vi "Initialize.vi"(8 "error in":errorcluster, 10 "InstanceName":string, 11 "Cycler Cluster - 24 Channel.lvclass":refnum<class "Cycler Cluster - 6 Channel.lvclass">) -> (0 "error out":errorcluster, 3 "output cluster":refnum<class "Cycler Cluster - 6 Channel.lvclass">)   [LabVIEW 2023, in "Cycler Cluster - 6 Channel.lvclass"]
uses:
  Cycler Cluster - 6 Channel.lvclass
  Cycler Cluster - 6 Channel.lvclass/Cycler Cluster - 6 Channel.ctl
  7d45be24-9a40-4f36-b3d1-14bc4134107c.vi
  1abf7531-339f-4e14-8fbe-02c4e44e8943.vi
  da48c8f8-b897-4dcf-9451-5b341042a248.vi
  f0f9fcd1-ad99-4552-afb1-31be6853704b.vi
  7d45be24-9a40-4f36-b3d1-14bc4134107c.vi/4bc1c15b-36ab-481f-b8dd-c64075ce723a.vi
  1abf7531-339f-4e14-8fbe-02c4e44e8943.vi/4bc1c15b-36ab-481f-b8dd-c64075ce723a.vi
  da48c8f8-b897-4dcf-9451-5b341042a248.vi/4bc1c15b-36ab-481f-b8dd-c64075ce723a.vi
  f0f9fcd1-ad99-4552-afb1-31be6853704b.vi/4bc1c15b-36ab-481f-b8dd-c64075ce723a.vi
  <vilib>/ADAS Replay HIL/AdasHilServices/AdasHilServices Fill In Error Info Ex.vi
  Utilities/Utilities.lvlib
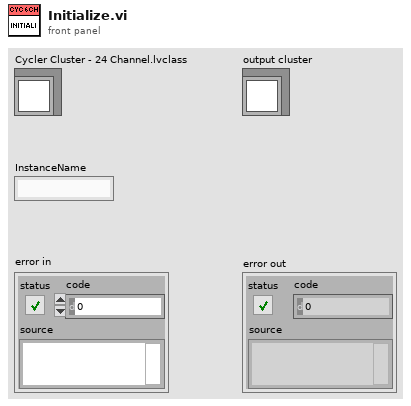
[diagram p1: front panel]
types:
  T1 = cluster{"OnOff.ACT":bool, "ErrorAcknowledge.ACT":bool, "IsoMeasurement.ACT":bool, "ParallelMode.ACT":bool}
  T2 = cluster{"OnOff.STS":i32, "Error.STS":i32, "Watchdog.STS":i32, "IsoMeasurement.STS":i32, "ParallelMode.STS":i32}
  T3 = cluster{"ErrorAcknowledge.ch01.ACT":bool, "OutputEnable.ch01.ACT":bool, "ControlMode.ch01.CTL":u16, "Voltage.ch01.SP":dbl, "VoltageMIN.ch01.SP":dbl, "VoltageMAX.ch01.SP":dbl, "VoltageGrad.ch01.SP":dbl, "Current.ch01.SP":dbl, "CurrentMIN.ch01.SP":dbl, "CurrentMAX.ch01.SP":dbl, "CurrentGrad.ch01.SP":dbl, "Power.ch01.SP":dbl, "Power.ch01.SP":dbl, "Power.ch01.SP":dbl, "PowerGrad.ch01.SP":dbl, "ParameterSet.ch01.CTL":i32}
  T4 = cluster{"Error.ch01.STS":i32, "OutputEnable.ch01.STS":i32, "ControlMode.ch01.STS":u16, "Voltage.ch01.AV":dbl, "Current.ch01.AV":dbl, "Power.ch01.AV":dbl, "VoltageNominal.ch01.AV":dbl, "CurrentNominal.ch01.AV":dbl, "PowerNominal.ch01.AV":dbl, "ParameterSet.ch01.STS":i32}
  T5 = cluster{"ErrorAcknowledge.ch02.ACT":bool, "OutputEnable.ch02.ACT":bool, "ControlMode.ch02.CTL":u16, "Voltage.ch02.SP":dbl, "VoltageMIN.ch02.SP":dbl, "VoltageMAX.ch02.SP":dbl, "VoltageGrad.ch02.SP":dbl, "Current.ch02.SP":dbl, "CurrentMIN.ch02.SP":dbl, "CurrentMAX.ch02.SP":dbl, "CurrentGrad.ch02.SP":dbl, "Power.ch02.SP":dbl, "PowerMIN.ch02.SP":dbl, "PowerMAX.ch02.SP":dbl, "PowerGrad.ch02.SP":dbl, "ParameterSet.ch02.CTL":i32}
  T6 = cluster{"Error.ch02.STS":i32, "OutputEnable.ch02.STS":i32, "ControlMode.ch02.STS":u16, "Voltage.ch02.AV":dbl, "Current.ch02.AV":dbl, "Power.ch02.AV":dbl, "VoltageNominal.ch02.AV":dbl, "CurrentNominal.ch02.AV":dbl, "PowerNominal.ch02.AV":dbl, "ParameterSet.ch02.STS":i32}
  T7 = cluster{"ErrorAcknowledge.ch03.ACT":bool, "OutputEnable.ch03.ACT":bool, "ControlMode.ch03.CTL":u16, "Voltage.ch03.SP":dbl, "VoltageMIN.ch03.SP":dbl, "VoltageMAX.ch03.SP":dbl, "VoltageGrad.ch03.SP":dbl, "Current.ch03.SP":dbl, "CurrentMIN.ch03.SP":dbl, "CurrentMAX.ch03.SP":dbl, "CurrentGrad.ch03.SP":dbl, "Power.ch03.SP":dbl, "PowerMIN.ch03.SP":dbl, "PowerMAX.ch03.SP":dbl, "PowerGrad.ch03.SP":dbl, "ParameterSet.ch03.CTL":i32}
  T8 = cluster{"Error.ch03.STS":i32, "OutputEnable.ch03.STS":i32, "ControlMode.ch03.STS":u16, "Voltage.ch03.AV":dbl, "Current.ch03.AV":dbl, "Power.ch03.AV":dbl, "VoltageNominal.ch03.AV":dbl, "CurrentNominal.ch03.AV":dbl, "PowerNominal.ch03.AV":dbl, "ParameterSet.ch03.STS":i32}
  T9 = cluster{"ErrorAcknowledge.ch04.ACT":bool, "OutputEnable.ch04.ACT":bool, "ControlMode.ch04.CTL":u16, "Voltage.ch04.SP":dbl, "VoltageMIN.ch04.SP":dbl, "VoltageMAX.ch04.SP":dbl, "VoltageGrad.ch04.SP":dbl, "Current.ch04.SP":dbl, "CurrentMIN.ch04.SP":dbl, "CurrentMAX.ch04.SP":dbl, "CurrentGrad.ch04.SP":dbl, "Power.ch04.SP":dbl, "PowerMIN.ch04.SP":dbl, "PowerMAX.ch04.SP":dbl, "PowerGrad.ch04.SP":dbl, "ParameterSet.ch04.CTL":i32}
  T10 = cluster{"Error.ch04.STS":i32, "OutputEnable.ch04.STS":i32, "ControlMode.ch04.STS":u16, "Voltage.ch04.AV":dbl, "Current.ch04.AV":dbl, "Power.ch04.AV":dbl, "VoltageNominal.ch04.AV":dbl, "CurrentNominal.ch04.AV":dbl, "PowerNominal.ch04.AV":dbl, "ParameterSet.ch04.STS":i32}
  T11 = cluster{"ErrorAcknowledge.ch05.ACT":bool, "OutputEnable.ch05.ACT":bool, "ControlMode.ch05.CTL":u16, "Voltage.ch05.SP":dbl, "VoltageMIN.ch05.SP":dbl, "VoltageMAX.ch05.SP":dbl, "VoltageGrad.ch05.SP":dbl, "Current.ch05.SP":dbl, "CurrentMIN.ch05.SP":dbl, "CurrentMAX.ch05.SP":dbl, "CurrentGrad.ch05.SP":dbl, "Power.ch05.SP":dbl, "PowerMIN.ch05.SP":dbl, "PowerMAX.ch05.SP":dbl, "PowerGrad.ch05.SP":dbl, "ParameterSet.ch05.CTL":i32}
  T12 = cluster{"Error.ch05.STS":i32, "OutputEnable.ch05.STS":i32, "ControlMode.ch05.STS":u16, "Voltage.ch05.AV":dbl, "Current.ch05.AV":dbl, "Power.ch05.AV":dbl, "VoltageNominal.ch05.AV":dbl, "CurrentNominal.ch05.AV":dbl, "PowerNominal.ch05.AV":dbl, "ParameterSet.ch05.STS":i32}
  T13 = cluster{"ErrorAcknowledge.ch06.ACT":bool, "OutputEnable.ch06.ACT":bool, "ControlMode.ch06.CTL":u16, "Voltage.ch06.SP":dbl, "VoltageMIN.ch06.SP":dbl, "VoltageMAX.ch06.SP":dbl, "VoltageGrad.ch06.SP":dbl, "Current.ch06.SP":dbl, "CurrentMIN.ch06.SP":dbl, "CurrentMAX.ch06.SP":dbl, "CurrentGrad.ch06.SP":dbl, "Power.ch06.SP":dbl, "PowerMIN.ch06.SP":dbl, "PowerMAX.ch06.SP":dbl, "PowerGrad.ch06.SP":dbl, "ParameterSet.ch06.CTL":i32}
  T14 = cluster{"Error.ch06.STS":i32, "OutputEnable.ch06.STS":i32, "ControlMode.ch06.STS":u16, "Voltage.ch06.AV":dbl, "Current.ch06.AV":dbl, "Power.ch06.AV":dbl, "VoltageNominal.ch06.AV":dbl, "CurrentNominal.ch06.AV":dbl, "PowerNominal.ch06.AV":dbl, "ParameterSet.ch06.STS":i32}
  T15 = cluster{"ErrorAcknowledge.ch06.ACT":bool, "OutputEnable.ch06.ACT":bool, "ControlMode.ch06.CTL":u16, "Voltage.ch06.SP":dbl, "VoltageMIN.ch06.SP":dbl, "VoltageMAX.ch06.SP":dbl, "VoltageGrad.ch06.SP":dbl, "Current.ch06.SP":dbl, "CurrentMIN.ch06.SP":dbl, "CurrentMAX.ch06.SP":dbl, "CurrentGrad.ch06.SP":dbl, "Power.ch06.SP":dbl, "PowerMIN.ch06.SP":dbl, "PowerMAX.ch06.SP":dbl, "PowerGrad.ch06.SP":dbl, "ParameterSet.ch06.CTL":i32}[]
  T16 = cluster{"Error.ch06.STS":i32, "OutputEnable.ch06.STS":i32, "ControlMode.ch06.STS":u16, "Voltage.ch06.AV":dbl, "Current.ch06.AV":dbl, "Power.ch06.AV":dbl, "VoltageNominal.ch06.AV":dbl, "CurrentNominal.ch06.AV":dbl, "PowerNominal.ch06.AV":dbl, "ParameterSet.ch06.STS":i32}[]
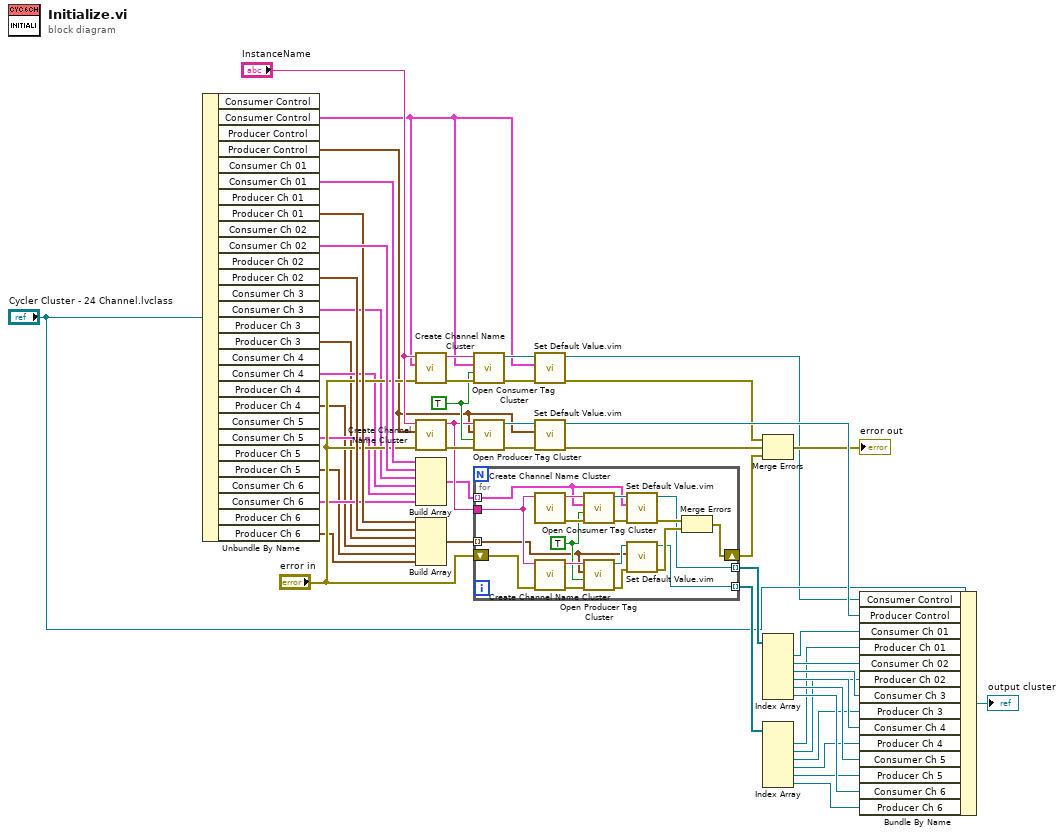
[diagram p0: block diagram]
diagram:
  w34 = TRUE ("Create if not found? (T)")
  n1 = Unbundle By Name("Cycler Cluster - 24 Channel.lvclass") -> ("Consumer Control"=w2:T1, "Producer Control"=w1:T2, "Consumer Ch 01"=w36:T3, "Producer Ch 01"=w32:T4, "Consumer Ch 02"=w35:T5, "Producer Ch 02"=w31:T6, "Consumer Ch 3"=w24:T7, "Producer Ch 3"=w20:T8, "Consumer Ch 4"=w23:T9, "Producer Ch 4"=w19:T10, "Consumer Ch 5"=w22:T11, "Producer Ch 5"=w18:T12, "Consumer Ch 6"=w21:T13, "Producer Ch 6"=w17:T14)  [unwired: 14 out]
  n2 = call "Create Channel Name Cluster.vi"("error in"="error in", "Cluster"=w2, "Instance Name"="InstanceName") -> ("error out"=w42:errorcluster, "Data Channel Name"=w49:string)  [unwired: 7 in]
  n3 = call "Create Channel Name Cluster.vi"("error in"="error in", "Cluster"=w1, "Instance Name"="InstanceName") -> ("error out"=w43:errorcluster, "Data Channel Name"=w33:string)  [unwired: 7 in]
  n4 = Build Array(w36, w35, w24, w23, w22, w21) -> (w3:T15)
  n5 = Build Array(w32, w31, w20, w19, w18, w17) -> (w30:T16)
  n6 = call "Open Consumer Tag Cluster.vi"("error in"=w42, "Create if not found? (T)"=w34, "Cluster"=w2, "Channel Name"=w49) -> ("error out"=w47:errorcluster, "ADAS HIL Channel"=w48:refnum<k21>)  [unwired: 6 in]
  n7 = call "Open Producer Tag Cluster.vi"("error in"=w43, "Create if not found? (T)"=w34, "Cluster"=w1, "Channel Name"=w33) -> ("error out"=w46:errorcluster, "ADAS HIL Channel"=w45:refnum<k21>)  [unwired: 6 in]
  n8 = for {
    tunnel: w33 -> [w58]
    tunnel: w3 -> [w50] mode=indexing
    tunnel: w30 -> [w51] mode=indexing
    shift-right: [w54] -> w28
    shift-left: "error in" -> [w57]
    tunnel: [w53] -> w26 mode=indexing
    tunnel: [w52] -> w12 mode=indexing
    w59 = TRUE ("Create if not found? (T)")
    n9 = call "Create Channel Name Cluster.vi"("Instance Name"=w58) -> ("error out"=w60:errorcluster, "Data Channel Name"=w67:string)  [unwired: 9 in]
    n10 = call "Create Channel Name Cluster.vi"("error in"=w57, "Instance Name"=w58) -> ("error out"=w61:errorcluster, "Data Channel Name"=w66:string)  [unwired: 8 in]
    n11 = call "Open Consumer Tag Cluster.vi"("error in"=w60, "Create if not found? (T)"=w59, "Cluster"=w50, "Channel Name"=w67) -> ("error out"=w64:errorcluster, "ADAS HIL Channel"=w65:refnum<k21>)  [unwired: 6 in]
    n12 = call "Open Producer Tag Cluster.vi"("error in"=w61, "Create if not found? (T)"=w59, "Cluster"=w51, "Channel Name"=w66) -> ("error out"=w63:errorcluster, "ADAS HIL Channel"=w62:refnum<k21>)  [unwired: 6 in]
    n13 = call "Set Default Value.vim"("error in"=w64, "Data in"=w50, "ADAS HIL Channel in"=w65) -> ("error out"=w55:errorcluster, "ADAS HIL Channel out"=w53:refnum<k21>)  [unwired: 7 in]
    n14 = call "Set Default Value.vim"("error in"=w63, "Data in"=w51, "ADAS HIL Channel in"=w62) -> ("error out"=w56:errorcluster, "ADAS HIL Channel out"=w52:refnum<k21>)  [unwired: 7 in]
    n15 = Merge Errors(w55, w56) -> (w54:errorcluster)
  }
  n16 = call "Set Default Value.vim"("error in"=w47, "Data in"=w2, "ADAS HIL Channel in"=w48) -> ("error out"=w41:errorcluster, "ADAS HIL Channel out"=w4:refnum<k21>)  [unwired: 7 in]
  n17 = call "Set Default Value.vim"("error in"=w46, "Data in"=w1, "ADAS HIL Channel in"=w45) -> ("error out"=w40:errorcluster, "ADAS HIL Channel out"=w44:refnum<k21>)  [unwired: 7 in]
  n18 = Merge Errors(w41, w40, w28) -> (→"error out":errorcluster)
  n19 = Index Array(array=w26) -> (element #1=w27:refnum<k21>, element #2=w25:refnum<k21>, element #3=w16:refnum<k21>, element #4=w15:refnum<k21>, element #5=w14:refnum<k21>, element #6=w13:refnum<k21>)  [unwired: 6 in]
  n20 = Index Array(array=w12) -> (element #1=w11:refnum<k21>, element #2=w10:refnum<k21>, element #3=w9:refnum<k21>, element #4=w8:refnum<k21>, element #5=w7:refnum<k21>, element #6=w6:refnum<k21>)  [unwired: 6 in]
  n21 = Bundle By Name(cluster="Cycler Cluster - 24 Channel.lvclass", "Consumer Control"=w4, "Producer Control"=w44, "Consumer Ch 01"=w27, "Producer Ch 01"=w11, "Consumer Ch 02"=w25, "Producer Ch 02"=w10, "Consumer Ch 3"=w16, "Producer Ch 3"=w9, "Consumer Ch 4"=w15, "Producer Ch 4"=w8, "Consumer Ch 5"=w14, "Producer Ch 5"=w7, "Consumer Ch 6"=w13, "Producer Ch 6"=w6) -> (→"output cluster":refnum<class "Cycler Cluster - 6 Channel.lvclass">)
